vi "Build Right Click Menu.vi"(8 "error in (no error)":errorcluster, 9 "Return Notifier":refnum<notifier>, 10 "Menu Click Data":T1, 11 "Main Display in":refnum<class "Main Display.lvclass">) -> (0 "error out":errorcluster, 3 "Main Display out":refnum<class "Main Display.lvclass">)   [LabVIEW 2016, in "Assert API Components.lvlib" / "Assert Display.lvlib" / "Main Display.lvlib" / "Main Display.lvclass"]
uses:
  Main Display.lvclass
  Menu Click Data.ctl
  <vilib>/Utility/miscctls.llb/LVPoint32TypeDef.ctl
  Main Display.lvclass/Main Display.ctl
  Display Configurations/Base Display Configuration.lvclass
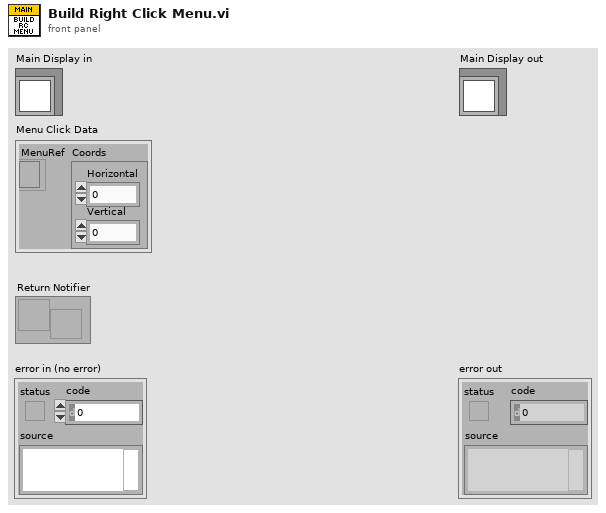
[diagram p1: front panel]
types:
  T1 = typedef "Menu Click Data.ctl" = cluster{"MenuRef":refnum<k9>, "Coords":T2}
  T2 = typedef "LVPoint32TypeDef.ctl" = cluster{"Horizontal":i32, "Vertical":i32}
  T3 = typedef "LVRowAndColumnTypeDef.ctl" = cluster{"Row":i32, "Column":i32}
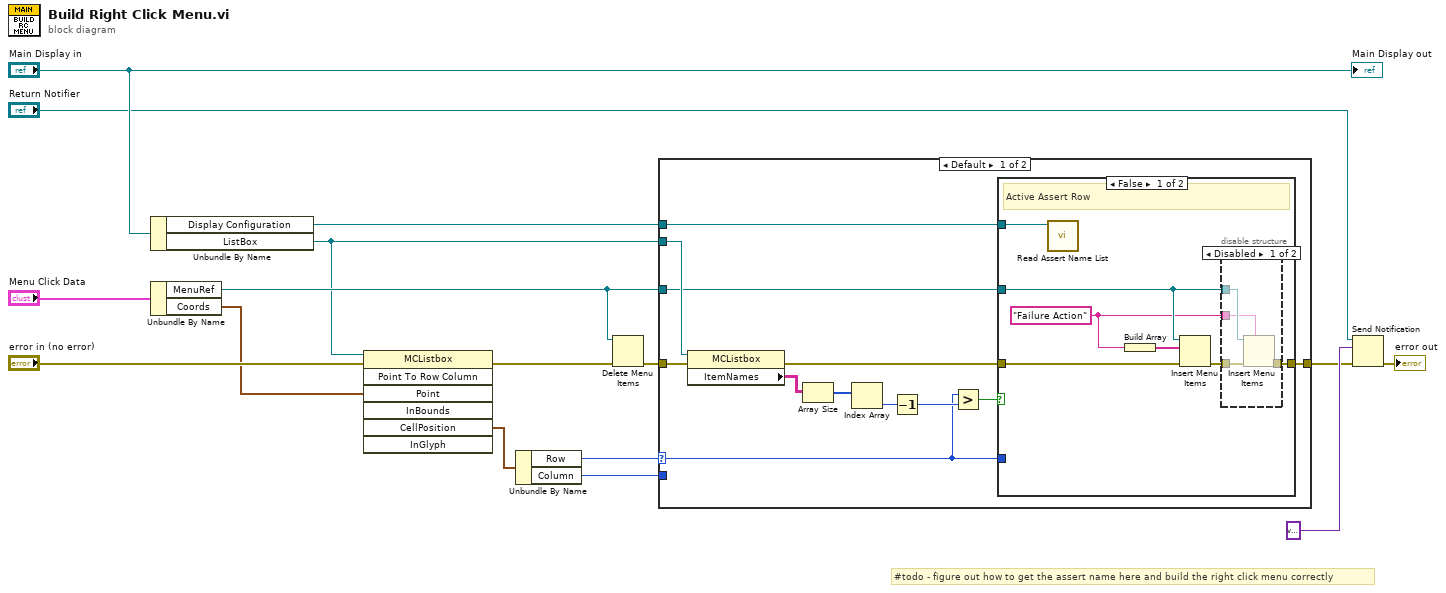
[diagram p0: block diagram]
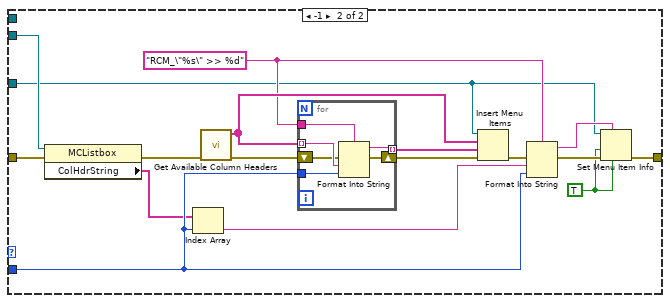
[diagram p4: hidden frame]
diagram:
  # "#todo - figure out how to get the assert name here and build the right click menu correctly"
  n1 = Unbundle By Name("Main Display in") -> ("Display Configuration"=w1:refnum<class "Base Display Configuration.lvclass">, "ListBox"=w2:refnum<vi>)
  n2 = Unbundle By Name("Menu Click Data") -> ("MenuRef"=w3:refnum<k9>, "Coords"=w4:T2)
  n3 = invoke on="Invoke Node" class="MCListbox" method="Point To Row Column"(reference=w2, error in="error in (no error)", "Point"=w4) -> (error out=w7:errorcluster, "CellPosition"=w11:T3)  [unwired: 4 in, 5 out]
  n4 = Unbundle By Name(w11) -> ("Row"=w9:i32, "Column"=w8:i32)
  n5 = Delete Menu Items(6:w7, 9:w3) -> (0:w10:errorcluster)  [unwired: 2 in, 1 out]
  n6 = case shown="Default" w9 {
    selector: w9 -> [w20 _]
    tunnel: [w18 w48] -> w5
    tunnel: w3 -> [w19 w41]
    tunnel: w10 -> [w28 w44]
    tunnel: w8 -> [_ w46]
    tunnel: w2 -> [w27 w45]
    tunnel: w1 -> [w17 _]
    frame Default {
      n7 = property class="MCListbox"(reference=w27, error in=w28) -> (error out=w21:errorcluster, "ItemNames"=w26:string[][])  [unwired: 1 out]
      n8 = Array Size(array=w26) -> (size(s)=w25:i32[])
      n9 = Index Array(array=w25) -> (element=w24:i32)  [unwired: 1 in]
      n10 = Decrement(x=w24) -> (x-1=w23:i32)
      n11 = Greater?(x=w20, y=w23) -> (0:w22:bool)
      n12 = case shown="False" w22 {
        tunnel: w21 -> [w35 w40]
        tunnel: w20 -> [_ _]
        tunnel: w19 -> [w31 _]
        tunnel: [w32 w40] -> w18
        tunnel: w17 -> [w29 _]
        frame False {
          w30 = "Failure Action"
          # "Active Assert Row"
          n13 = call "Read Assert Name List.vi"("Base Display Configuration in"=w29) -> ()  [unwired: 10 in, 1 out]
          n14 = Build Array(w30) -> (w33:string[])
          n15 = Insert Menu Items(6:w35, 8:w33, 9:w31) -> (0:w34:errorcluster)  [unwired: 3 in, 2 out]
          n16 = disable-structure shown="Disabled" {
            disable-tunnel: w34 -> [w39 _]
            disable-tunnel: [w38 _] -> w32
            disable-tunnel: w31 -> [w37 _]
            disable-tunnel: w30 -> [w36 _]
            frame Disabled {
              n17 = Insert Menu Items(5:w36, 6:w39, 9:w37) -> (0:w38:errorcluster)  [unwired: 3 in, 2 out]
            }
            frame Enabled {
            }
          }
        }
        frame True {
          # "Not clicked on an active assert row"
        }
      }
    }
    frame -1 {
      w47 = TRUE ("enabled")
      w52 = "RCM_\"%s\" >> %d" ("format string")
      n18 = property class="MCListbox"(reference=w45, error in=w44) -> (error out=w42:errorcluster, "ColHdrString"=w43:string[])  [unwired: 1 out]
      n19 = Index Array(array=w43, index=w46) -> (element=w51:string)
      n20 = call "Get Available Column Headers.vi"("error in (no error)"=w42) -> ("error out"=w55:errorcluster, "Available Column Headers"=w57:string[])  [unwired: 9 in]
      n21 = for {
        tunnel: w57 -> [w63] mode=indexing
        tunnel: [w62] -> w49 mode=indexing
        shift-right: [w60] -> w54
        shift-left: w55 -> [w61]
        tunnel: w52 -> [w59]
        tunnel: w46 -> [w58]
        n22 = Format Into String(format string=w59, error in=w61, w63, w58) -> (resulting string=w62:string, error out=w60:errorcluster)  [unwired: 1 in]
      }
      n23 = Insert Menu Items(6:w54, 7:w49, 8:w57, 9:w41) -> (0:w56:errorcluster)  [unwired: 2 in, 2 out]
      n24 = Format Into String(format string=w52, error in=w56, w51, w46) -> (resulting string=w50:string, error out=w53:errorcluster)  [unwired: 1 in]
      n25 = Set Menu Item Info(6:w47, 7:w50, 8:w53, 9:w47, 11:w41) -> (0:w48:errorcluster)  [unwired: 2 in, 1 out]
    }
  }
  n26 = Send Notification(notification=variant, notifier="Return Notifier", error in (no error)=w5) -> (error out=→"error out":errorcluster)  [unwired: 1 out]
  "Main Display out" <- "Main Display in"
